vi "Phase Rotation.vi"() -> ()   [LabVIEW 2018]
panel:
  in  "Stop Button":bool
  in  "Angle":dbl(slide)=-0.21212121212121193 scale=-3.0..3.0
  out "Waveform Graph":waveform(dbl)[](graph)=[{"t0"=timestamp(3643658336.8902287 s since 1904-01-01), "dt"=1.0, "Y"=array[1605 elements], "attributes"=variant("Configuration"=variant(string "[Configuration]\nConfiguration.Points per sine wave = \"68\"\nConfiguration.Rate = \"4080032.0171\"\nConfiguration.Re-name channels.<size(s)> = \"2\"\nConfiguration.Re-name channels 0 = \"V2\"\nConfiguration.Re-name channels 1 = \"I2\"\nConfiguration.Active channels = \"0:1\"\nConfiguration.Ranges = \"<size(s)=2> 6.0000000000 6.0000000000\"\nConfiguration.Sync on trigger = \"FALSE\"\nConfiguration.R-Q = \"FALSE\""), "NI_ChannelName"=variant(string "V2 X"), "NI_ExpTimeStamp"=variant(timestamp timestamp(3643658336.8902287 s since 1904-01-01)), "NI_UnitDescription"=variant(string "V"))}, {"t0"=timestamp(3643658336.8902287 s since 1904-01-01), "dt"=1.0, "Y"=array[1605 elements], "attributes"=variant("Configuration"=variant(string "[Configuration]\nConfiguration.Points per sine wave = \"68\"\nConfiguration.Rate = \"4080032.0171\"\nConfiguration.Re-name channels.<size(s)> = \"2\"\nConfiguration.Re-name channels 0 = \"V2\"\nConfiguration.Re-name channels 1 = \"I2\"\nConfiguration.Active channels = \"0:1\"\nConfiguration.Ranges = \"<size(s)=2> 6.0000000000 6.0000000000\"\nConfiguration.Sync on trigger = \"FALSE\"\nConfiguration.R-Q = \"FALSE\""), "NI_ChannelName"=variant(string "V2 Y"), "NI_ExpTimeStamp"=variant(timestamp timestamp(3643658336.8902287 s since 1904-01-01)), "NI_UnitDescription"=variant(string "V"))}, {"t0"=timestamp(3643658336.8902287 s since 1904-01-01), "dt"=1.0, "Y"=array[1605 elements], "attributes"=variant("Configuration"=variant(string "[Configuration]\nConfiguration.Points per sine wave = \"68\"\nConfiguration.Rate = \"4080032.0171\"\nConfiguration.Re-name channels.<size(s)> = \"2\"\nConfiguration.Re-name channels 0 = \"V2\"\nConfiguration.Re-name channels 1 = \"I2\"\nConfiguration.Active channels = \"0:1\"\nConfiguration.Ranges = \"<size(s)=2> 6.0000000000 6.0000000000\"\nConfiguration.Sync on trigger = \"FALSE\"\nConfiguration.R-Q = \"FALSE\""), "NI_ChannelName"=variant(string "V2 X"), "NI_ExpTimeStamp"=variant(timestamp timestamp(3643658336.8902287 s since 1904-01-01)), "NI_UnitDescription"=variant(string "V"))}, {"t0"=timestamp(0 s since 1904-01-01), "dt"=1.0, "Y"=array[1605 elements]}]
  in  "Channels":string[](array[string])=["V2 X", "V2 Y"]
  in  "Group":string="p"
  in  "File Path Control":path
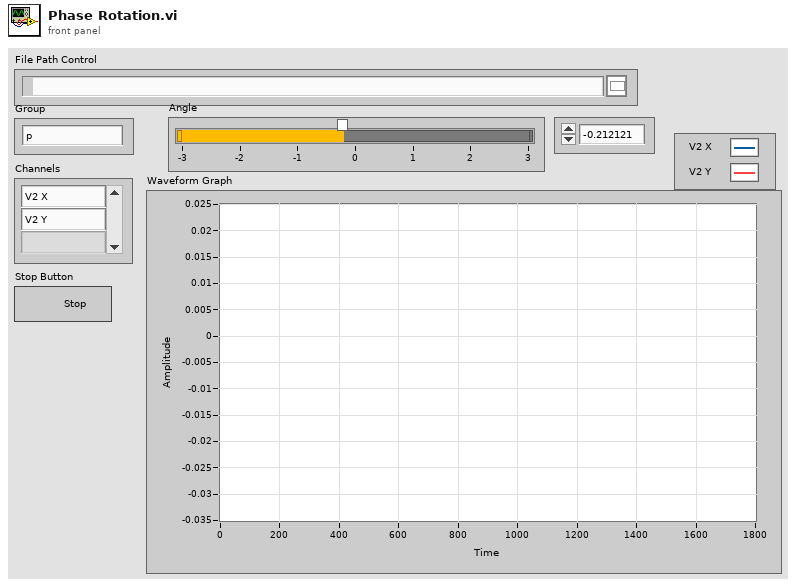
[diagram p1: front panel]
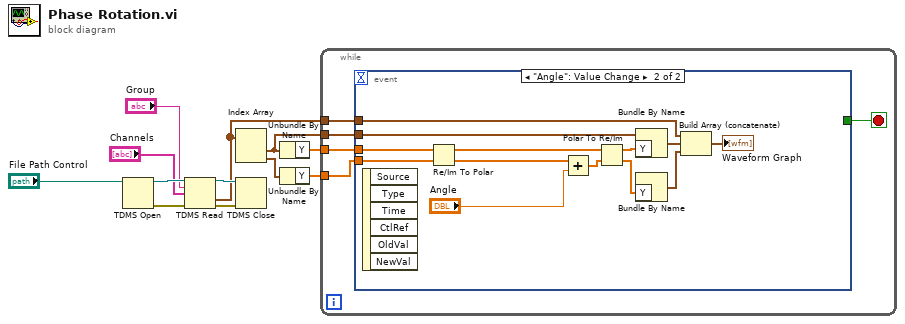
[diagram p0: block diagram]
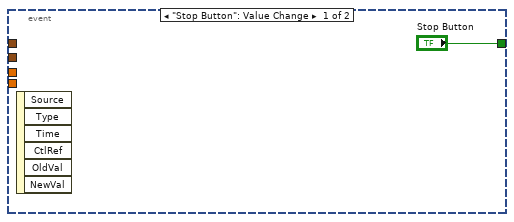
[diagram p2: hidden frame]
diagram:
  n1 = TDMS Open(11:"File Path Control") -> (0:w10:errorcluster, 3:w11:refnum<k34>)  [unwired: 6 in]
  n2 = TDMS Read(0:w11, 5:"Group", 7:"Channels", 11:w10) -> (4:w7:refnum<k34>, 10:w4:waveform(dbl)[], 15:w6:errorcluster)  [unwired: 4 in, 3 out]
  n3 = Index Array(array=w4) -> (element #1=w3:waveform(dbl), element #2=w5:waveform(dbl))  [unwired: 2 in]
  n4 = TDMS Close(8:w6, 11:w7) -> ()  [unwired: 2 out]
  n5 = Unbundle By Name(w3) -> ("Y"=w1:dbl[])
  n6 = Unbundle By Name(w5) -> ("Y"=w2:dbl[])
  n7 = while {
    tunnel: w4 -> [w16]
    tunnel: w3 -> [w15]
    tunnel: w2 -> [w14]
    tunnel: w1 -> [w13]
    stop <- w17 stop-if-true
    n8 = event shown="[1] \"Angle\": Value Change" {
      selector: _ -> [_ _]
      dyn-events: _ -> [_ _]
      timeout: _ -> [_ _]
      tunnel: ["Stop Button" _] -> w17
      tunnel: w16 -> [_ w24]
      tunnel: w15 -> [_ w23]
      tunnel: w14 -> [_ w22]
      tunnel: w13 -> [_ w21]
      event "Stop Button": Value Change {
        n9 = event-data() -> ()  [unwired: 1 in, 6 out]
      }
      event "Angle": Value Change {
        n10 = event-data() -> ()  [unwired: 1 in, 6 out]
        n11 = Re/Im To Polar(2:w22, 3:w21) -> (0:w25:dbl[], 1:w27:dbl[])
        n12 = Add(x=w25, y="Angle") -> (x+y=w26:dbl[])
        n13 = Polar To Re/Im(2:w26, 3:w27) -> (0:w29:dbl[], 1:w28:dbl[])
        n14 = Bundle By Name(cluster=w23, "Y"=w28) -> (w30:waveform(dbl))
        n15 = Bundle By Name("Y"=w29) -> (w31:waveform(dbl))  [unwired: 1 in]
        n16 = Build Array (concatenate)(w24, w30, w31) -> (→"Waveform Graph":waveform(dbl)[])
      }
    }
  }
